vi "Read Device and Session.vi"(8 "error in (no error)":errorcluster, 11 "SLSC Switch in":refnum<class "SLSC Switch.lvclass">) -> (0 "error out":errorcluster, 1 "device":refnum<k21>, 2 "session":refnum<k21>, 3 "SLSC Switch out":refnum<class "SLSC Switch.lvclass">)   [LabVIEW 2015]
uses:
  SLSC Switch.lvclass
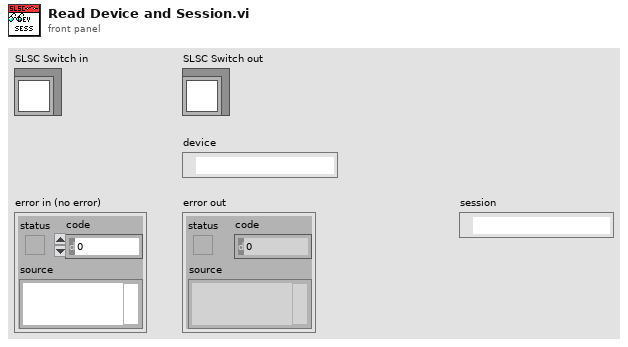
[diagram p1: front panel]
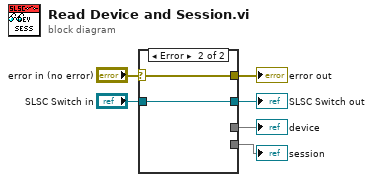
[diagram p0: block diagram]
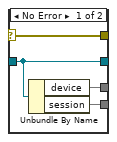
[diagram p2: hidden frame]
diagram:
  n1 = case shown="Error" "error in (no error)" {
    selector: "error in (no error)" -> [w10 w11]
    tunnel: [w10 w11] -> w5
    tunnel: [w9 w12] -> w3
    tunnel: "SLSC Switch in" -> [w9 w12]
    tunnel: [w8 _] -> w2
    tunnel: [w7 _] -> w1
    frame No Error {
      n2 = Unbundle By Name(w9) -> ("device"=w8, "session"=w7)
    }
    frame Error {
    }
  }
  "error out" <- w5
  "SLSC Switch out" <- w3
  "device" <- w2
  "session" <- w1
